vi "Intan_StreamData_128ch_parallelLoop_noEventStruct.vi"(0 "VISA resource name":refnum<visa-resource-name>, 1 "refnum in":refnum<file>, 3 "stop streaming":bool, 4 "Save Binary Data":bool, 5 "error in":errorcluster, 7 "byte order":T5(ring)=enum."little-endian", 8 "hdr fpath":path, 9 "MaxStreamChans":u16=32, 11 "DT_scale (sec)":dbl=0.01, 12 "aux file ref num":refnum<file>, 14 "save aux file":bool) -> (6 "N data scans to read (VISA)":i32=20, 10 "Nbytes VISA read":u32, 13 "VISA read iter":i32, 19 "error out":errorcluster)   [LabVIEW 2020]
doc: "Stream data to disk and user friendly display. Data is scaled and filtered prior to display.\n\nThis VI uses parallel while loop architecture: 1 loop reads from serial stream and saves raw bytes to disk; the other loop processes the data in chunk, scaling and filtering, then displays."
uses:
  zip_swcircularbuffer1_0_19b/Circular Buffer/Controls/Circular Buffer Status.ctl
  zip_swcircularbuffer1_0_19b/Circular Buffer/Controls/Circular Buffer Operations.ctl
  <vilib>/Utility/error.llb/DialogType.ctl
  <vilib>/Analysis/baseanly.llb/Mean (DBL).vi
  zip_swcircularbuffer1_0_19b/Circular Buffer/Instance VIs/Circular Buffer(1D U16).vi
  zip_swcircularbuffer1_0_19b/Circular Buffer/Circular Buffer.lvlib
  <vilib>/Analysis/NI_AALBase.lvlib
panel:
  out "A+B+C+D chans":i32[](array[numeric])
  out "C+D chans":i32[](array[numeric])
  out "Dchans":i32[](array[numeric])
  out "Cchans":i32[](array[numeric])
  out "ADXL/Vflex/Vdd Stream":dbl[][](graph)
  out "A+B chans":i32[](array[numeric])
  out "Bchans":i32[](array[numeric])
  out "Achans":i32[](array[numeric])
  in  "Tab Control":T1(tab)
  in  "Update Channels":bool
  in  "Accel/Vdd/Vflex":i32[](listbox)
  in  "stop logging":bool
  in  "DisplayScale (uV/div)":u16(ring)=1 items=["6400", "3200", "1600", "800", "400", "200", "100", "50", "25"]
  in  "offset factor":dbl=1.0
  in  "Filter settings":T2={"LP Filter On/Off"=TRUE, "LP Cutoff (Hz)"=40.0, "HP Filter On/Off"=TRUE, "HP Cutoff (Hz)"=0.5, "Bandstop On/Off"=TRUE, "fl Cutoff (Hz)"=48.0, "fh Cutoff (Hz) "=52.0}
  out "Save status":bool
  out "non integer read":bool
  out "display iter":i32
  out "% buffer full":dbl(slide) scale=0.0..100.0
  in  "Ring Buffer Size":T3={"Samples per Channel"=640000, "Channels"=0}
  out "buffer underflow":bool
  out "Buffer Status  (read)":T4
  out "buffer overflow":bool
  out "Buffer Status (write)":T4
  in  "Center Traces":bool
  in  "Amplifier Chans":i32[](listbox)=[1, 4, 13, 14, 15, 16, 17, 22]
  out "FS (Hz)":dbl
  in  "ChartDisplayLength (s)":dbl=5.0
  in  "Display Update interval (ms)":dbl=100.0
  in  "Buffer Read Interval (ms)":i16=100
  in  "ChanSelect":u16(ring)=7 items=["A chans (0-31)", "B chans (32-63)", "C chans (64-95)", "D chans (96-127)", "A+B chans (0-63)", "C+D chans (64-127)", "Free Select", "None"]
  out "Vdd amp (V)":dbl format="%0.1f"
  in  "bytes per data frame":i32=286
  in  "Nchans":i32=128
  in  "start stream (Teensy char)":string="s"
  in  "stop serial stream (Teensy char)":string="t"
  out "Text response":string
  out "aux_cmd_array":i32[][](array[numeric])
  out "binary data (from VISA read)":u16[](array[numeric])
  out "magicNum Out":i32[](array[numeric])
  in  "stop logging Teensy char":string="l"
  out "Vdd (V) out":dbl[](array[numeric])
  out "accel + flex + Vdd array":dbl[][](array[numeric])
  out "Vflex (V) out":dbl[](array[numeric])
  out "Data Frame Locked":string="circ buffer write:\nelement 0 ~= 73!"
  out "setscaleresult":dbl
  out "UpdateCode":i16
  out "xmax_init":dbl
  out "offset_init":dbl
  out "increment_init":dbl
  out "xmin_init":dbl
  out "NchansChanged":bool
  out "DispLengthChanged":bool
  out "XscaleRollover":bool
  out "error code out":i32 format="%0.0f"
  out "StopLoopsMaster":bool
  out "N_u16s  write to buf":i32
  out "Nelements to read from buf":dbl
  out "N data scans to display":u16=20
  out "YtxtLabelsAll":string[](array[string])
  out "bytes streaming per frame":u16
  out "requestBytes":dbl
  out "SerRead":string
  out "lengthCorStr":i32
  out "CorrectedSubstring":string
  out "NmissingFromFrame":i32
  out "bytesParsed":i32=148
  out "adxl size":i32[](array[numeric])
  out "intan size":i32[](array[numeric])
  out "ChanSelect(uint32)":u32[](array[numeric])
  out "ChanSelString":string
  out "NumChansNewStream":string
  out "Buffer Status Empty Buf":T4
  out "NumStreamingCluster":T6
  out "AmpsList":u16[](array[numeric])
  out "ClusterPropnod":T6
  out "ClusterLocalVar":T6
  out "Elements Remaining":i32
  out "termcharsReadBuffer":string
  out "termcharsCount":u32
  out "NumChansStreaming":i16
  out "initRead":string[](array[string])
  out "CircBufWrite":u16[](array[numeric])
  out "ReadCircBuf":u16[](array[numeric])
  out "subReadArray":u16[](array[numeric])
  out "corrected array":u16[](array[numeric])
  out "Nextraadded":i32
  out "extrareadelements":u16[](array[numeric])
  out "Picture":picture
  out "Intan Streaming Data":dbl[][](graph)
  # "Intan-Teensy Bioelectric Module: Data Stream and Visualization\n128 chan + ADXL"
  # "Data Streaming Frequency"
  # "Display Settings"
  # "Ring Buffer Status"
  # "1-D data stream \nreformatted  to 2-D"
  # "xscale controls"
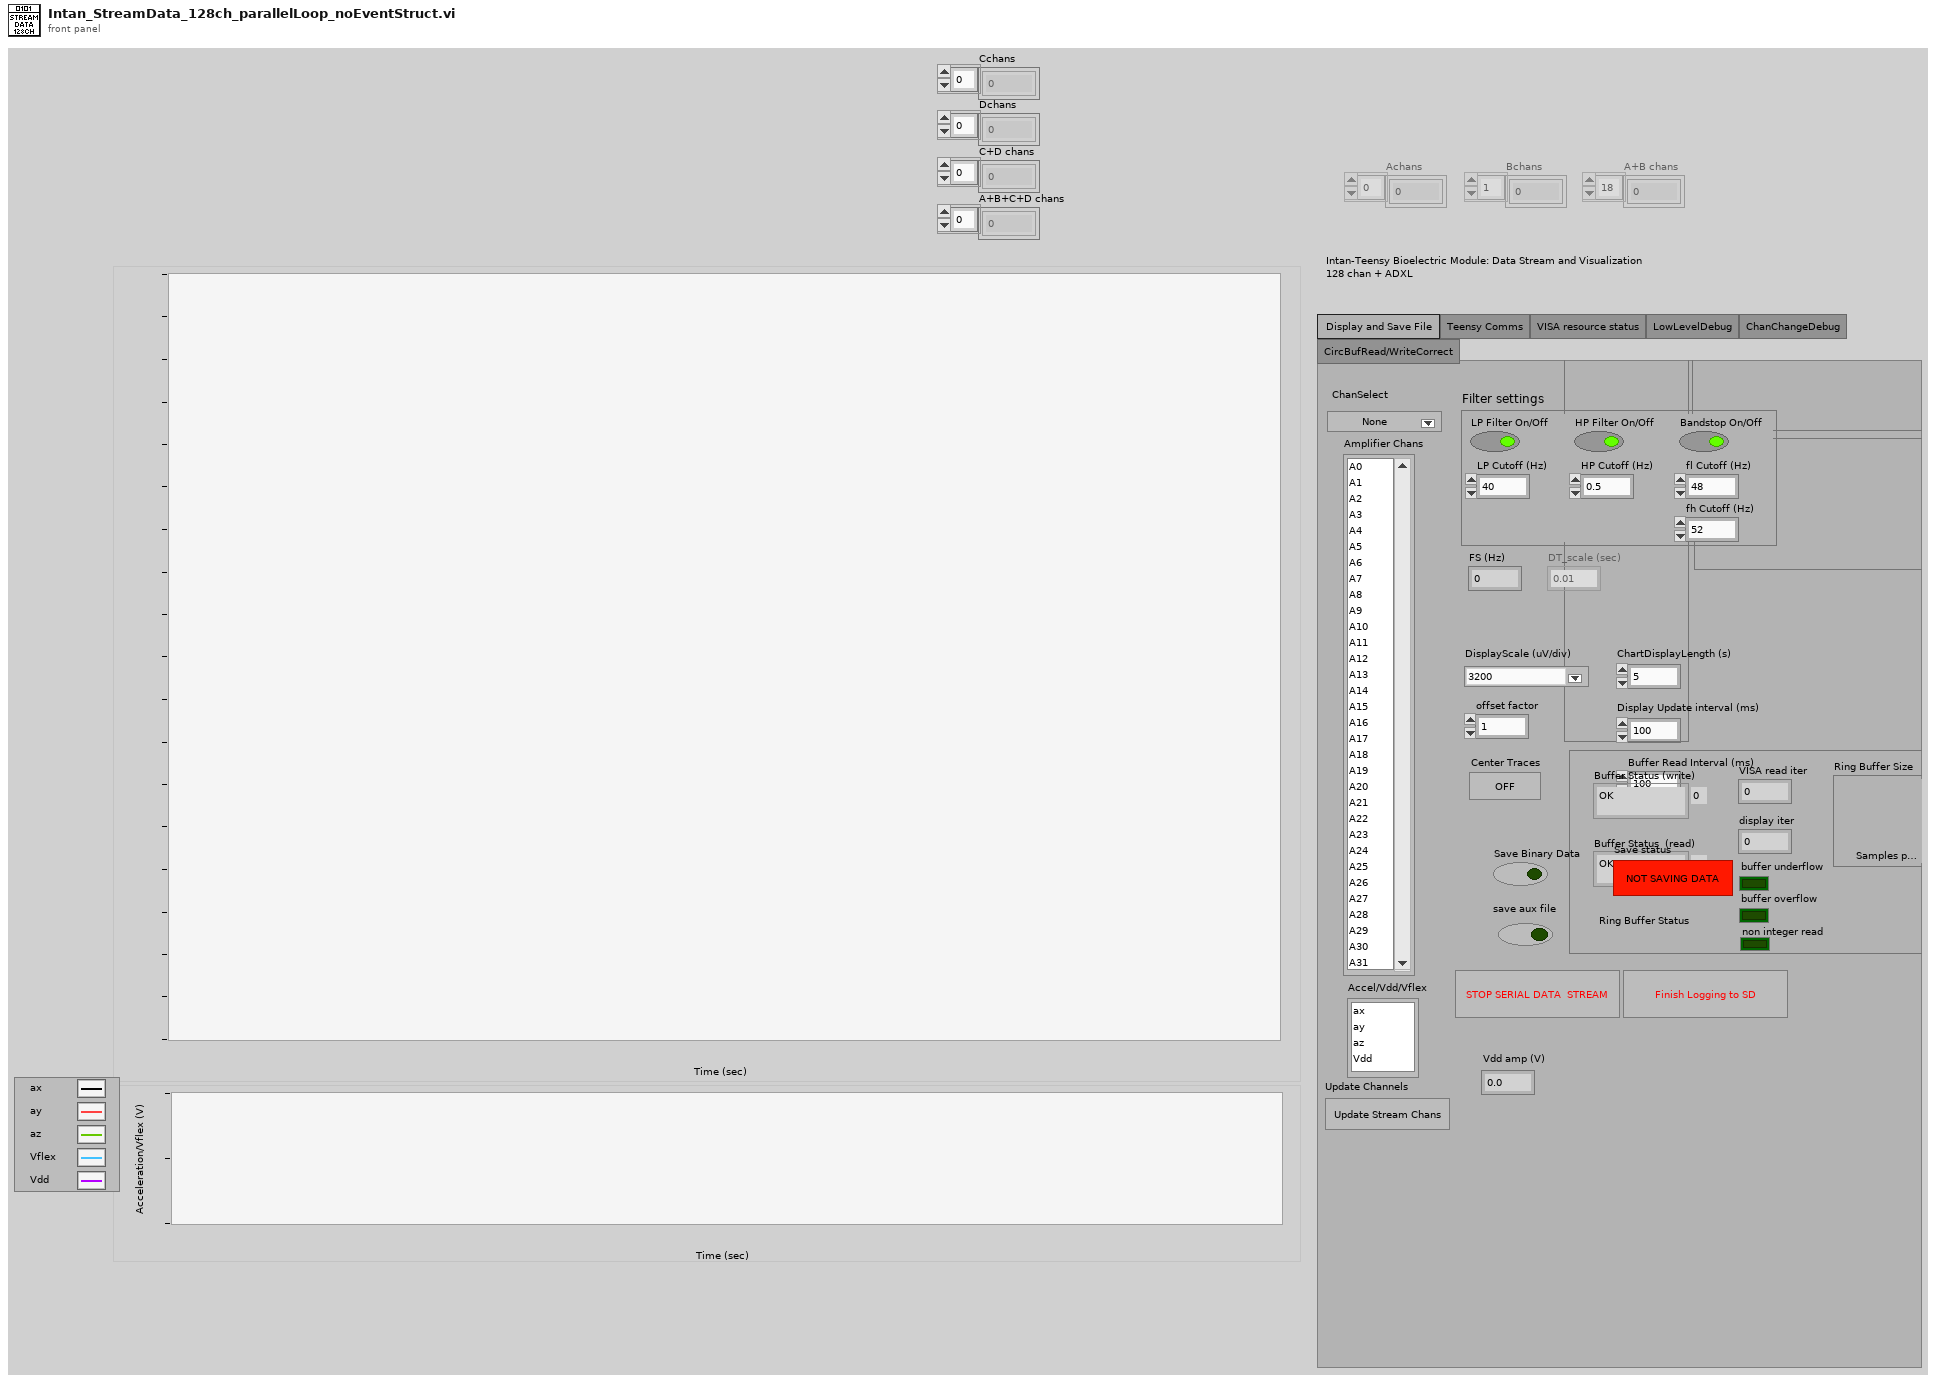
[diagram p1: front panel]
types:
  T1 = enum32{"Display and Save File ", "Teensy Comms", "VISA resource status", "LowLevelDebug", "ChanChangeDebug", "CircBufRead/WriteCorrect"}
  T2 = cluster{"LP Filter On/Off":bool, "LP Cutoff (Hz)":dbl, "HP Filter On/Off":bool, "HP Cutoff (Hz)":dbl, "Bandstop On/Off":bool, "fl Cutoff (Hz)":dbl, "fh Cutoff (Hz) ":dbl}
  T3 = cluster{"Samples per Channel":u32, "Channels":u32}
  T4 = typedef "Circular Buffer.lvlib/Circular Buffer Status.ctl" = enum16{"OK", "Overflow", "Underflow"}
  T5 = enum16{"big-endian, network order", "native, host order", "little-endian"}
  T6 = cluster{"NumChansStreaming":i16, "NumAmps":i32, "NumAccel":i32, "NumVdd":i32, "NumVflex":i32}
  T7 = enum8{"Enabled", "Disabled", "Disabled and Grayed Out"}
  T8 = typedef "Circular Buffer.lvlib/Circular Buffer Operations.ctl" = enum16{"Initialize", "Get Backlog", "Write", "Read (continuous)", "Read (most recent)"}
  T9 = typedef "LVRectTypeDef.ctl" = cluster{"Left":i16, "Top":i16, "Right":i16, "Bottom":i16}
  T10 = typedef "DialogType.ctl" = u16
  T11 = cluster{"XScale.Minimum":dbl, "XScale.Maximum":dbl, "XScale.Increment":dbl, "Nchannels":i32}
  T12 = cluster{"Maximum":dbl, dbl, dbl, dbl, dbl, dbl, "YscleMark":dbl, "Increment":dbl}
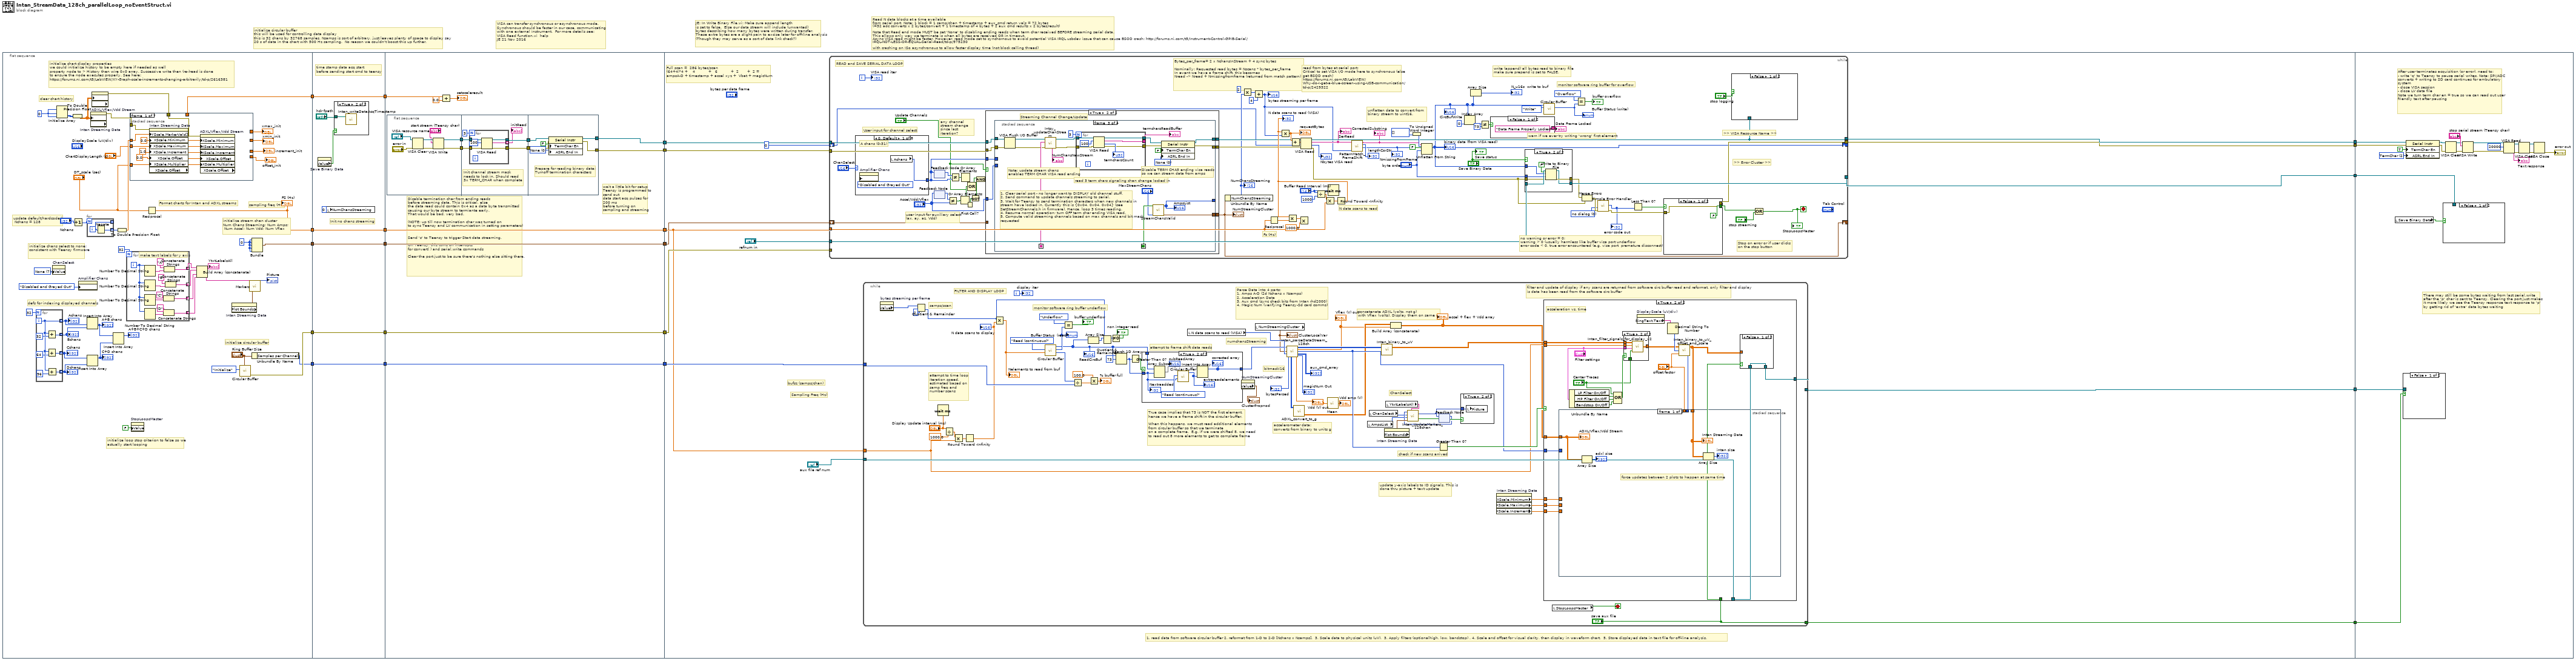
[diagram p0: block diagram]
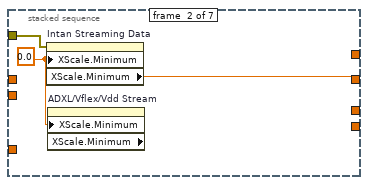
[diagram p2: hidden frame]
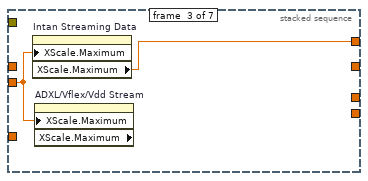
[diagram p3: hidden frame]
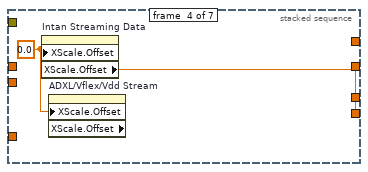
[diagram p4: hidden frame]
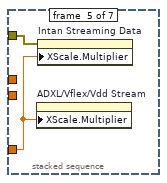
[diagram p5: hidden frame]
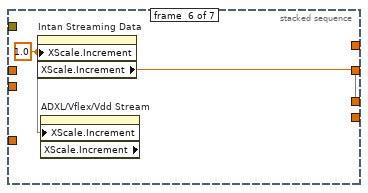
[diagram p6: hidden frame]
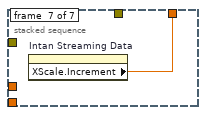
[diagram p7: hidden frame]
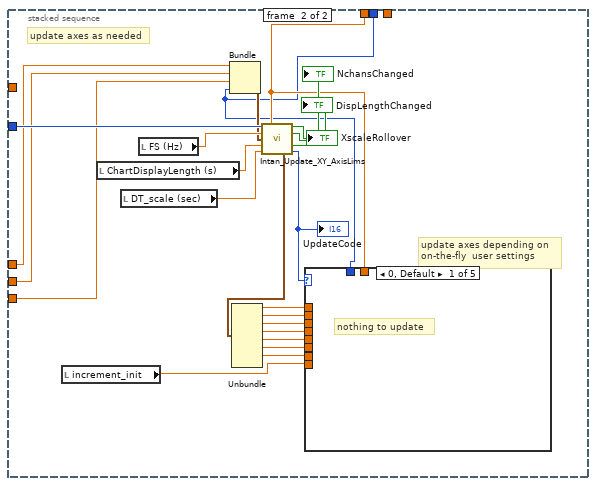
[diagram p12: hidden frame]
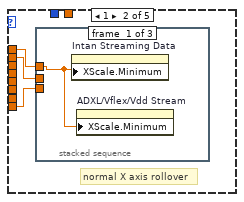
[diagram p13: hidden frame]
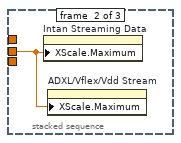
[diagram p14: hidden frame]
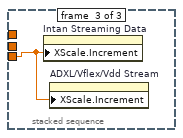
[diagram p15: hidden frame]
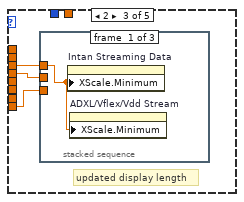
[diagram p16: hidden frame]
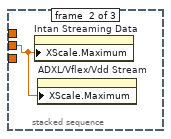
[diagram p17: hidden frame]
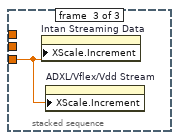
[diagram p18: hidden frame]
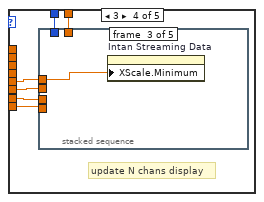
[diagram p19: hidden frame]
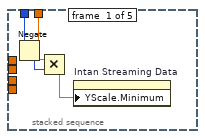
[diagram p20: hidden frame]
diagram:
  # "Read N data blocks at a time available\nfrom serial port. Note: 1 block = 1 samp/chan + timestamp + aux_cmd return vals = 72 bytes \n(=32 adc converts x 2 bytes/convert + 1 timestamp of 4 bytes + 2 aux cmd results x 2 bytes/result) \n\nNote that Read end mode MUST be set 'None' to disabling ending reads when term char received BEFORE streaming serial data.  \nThis allows only way we terminate is when all bytes are received OR in timeout.  \nAsync VISA read might be faster. However, read mode set to synchornous to avoid potential VISA IRQL usbdev issue that can cause BSOD crash: http://forums.ni.com/t5/Instrument-Control-GPIB-Serial/IRQL-NOT-LESS-OR-EQUAL-Serial-Read/td-p/975230\n\nwith crashing on ISo asynchronous to allow faster display time (not block calling thread)"
  # "initialize circular buffer\nthis will be used for controlling data display\nthis is 32 chans by 32768 samples. Nsamps is sort of arbitrary, just leaves plenty of space to display say\n20 s of data in the chart with 500 Hz sampling.  No reason we couldn't boost this up further."
  # "JE: In Write Binary File.vi: Make sure append length \nis set to false.  Else our data stream will include (unwanted)\nbytes describing how many bytes were written during transfer.\nThese extra bytes are a slight pain to excise later for off-line analysis\n(Though they may serve as a sort of data link check?)"
  # "VISA can transfer synchronous or asynchronous mode.\nSynchronous should be faster in our case, communicating\nwith one external instrument.  For more details see: \nVISA Read function.vi  help \nJE 21 Nov 2016"
  n1 = flat-sequence {
    tunnel: [w60] -> w13
    tunnel: [w58] -> w11
    tunnel: [w54] -> w9
    tunnel: [w43] -> w7
    tunnel: [w25] -> w5
    tunnel: w13 -> [w113]
    tunnel: [w113] -> w12
    tunnel: w11 -> [w112]
    tunnel: [w112] -> w10
    tunnel: w9 -> [w111]
    tunnel: [w111] -> w8
    tunnel: w7 -> [w110]
    tunnel: [w110] -> w6
    tunnel: w5 -> [w106]
    tunnel: [w106] -> w4
    tunnel: [w127] -> w19
    tunnel: w12 -> [w127]
    tunnel: [w126] -> w18
    tunnel: w10 -> [w126]
    tunnel: [w125] -> w17
    tunnel: w8 -> [w125]
    tunnel: w6 -> [w124]
    tunnel: w4 -> [w121]
    tunnel: [w121] -> w3
    tunnel: [w115] -> w2
    tunnel: [w116] -> w1
    tunnel: [w164] -> w21
    tunnel: [w165] -> w20
    tunnel: w19 -> [w163]
    tunnel: w18 -> [w162]
    tunnel: w17 -> [w161]
    tunnel: [w160] -> w16
    tunnel: [w158] -> w15
    tunnel: [w157] -> w14
    tunnel: w3 -> [w156]
    tunnel: w2 -> [w154]
    tunnel: w1 -> [w155]
    tunnel: w21 -> [w498]
    tunnel: w20 -> [w511]
    tunnel: w16 -> [w493]
    tunnel: w15 -> [w492]
    tunnel: w14 -> [w491]
    frame #0 {
      w24 = u16 7 items=["A chans (0-31)", "B chans (32-63)", "C chans (64-95)", "D chans (96-127)", "A+B chans (0-63)", "C+D chans (64-127)", "Free Select", "None"] ("ChanSelect")
      w22 = i16 0
      w53 = 0 ("Dimension Size")
      # "initialize chans select to none; consistent with Teensy firmware"
      # "initialize stream chan cluster\nNum Chans Streaming; Num Amps;\n Num Accel; Num Vdd; Num Vflex"
      # "initialize circular buffer"
      # "Format charts for Intan and ADXL streams"
      # "defs for indexing displayed channels"
      # "update default/hardcoded\n Nchans = 128"
      # "clear chart history"
      # "initialize loop stop criterion to false so we\nactually start looping"
      # "sampling freq (Hz)"
      # "initialize chart display properties\nwe could initialize history to be empty here if needed as well\nproperty node to > History then wire 0x0 array. Successive write then (re-)read is done\nto ensure the node executes properly. See here:\nhttps://forums.ni.com/t5/LabVIEW/XY-Graph-scale-increments-changing-arbitrarily/td-p/2616381"
      n2 = for {
        N: 32 -> [_]
        tunnel: [w68] -> w35 mode=indexing
        tunnel: [w69] -> w34 mode=indexing
        tunnel: [w65] -> w33 mode=indexing
        tunnel: [w64] -> w32 mode=indexing
        i -> [w68]
        n3 = Add(x=w68, y=32) -> (x+y=w69:i32)
        n4 = Add(x=w68, y=64) -> (x+y=w65:i32)
        n5 = Add(x=w68, y=96) -> (x+y=w64:i32)
      }
      "Achans" <- w35
      "Bchans" <- w34
      "Cchans" <- w33
      "Dchans" <- w32
      n6 = property on="ChanSelect" class="Ring (strict)"("Value"=w24) -> ()  [unwired: 2 in, 2 out]
      n7 = Initialize Array(w53, w53, w53) -> (w52:i32[][])
      n8 = To Double Precision Float(number=w52) -> (double precision float=w37:dbl[][])
      n9 = Increment(x="Nchans") -> (x+1=w62:i32)
      n10 = property on="Amplifier Chans" class="LstBox (strict)"("DisabledEnum"=T7."Disabled and Grayed Out" ("Disabled")) -> ()  [unwired: 2 in, 2 out]
      n11 = for {
        N: w62 -> [_]
        tunnel: [w105] -> w63 mode=indexing
        tunnel: [w104] -> _ mode=indexing
        i -> [w104]
        n12 = Negate(x=w104) -> (-x=w105:i32)
      }
      n13 = Insert Into Array(array=w35, new element=w34) -> (w31:i32[])  [unwired: 1 in]
      "A+B chans" <- w31
      n14 = Insert Into Array(array=w33, new element=w32) -> (w30:i32[])  [unwired: 1 in]
      "C+D chans" <- w30
      n15 = property on="Intan Streaming Data" class="WFChart (strict)" props=["History Data", "History Data"]("History Data"=w37) -> (error out=w50:errorcluster)  [unwired: 2 in, 2 out]
      n16 = property on="ADXL/Vflex/Vdd Stream" class="WFChart (strict)" props=["History Data", "History Data"]("History Data"=w37) -> (error out=w36:errorcluster)  [unwired: 2 in, 2 out]
      n17 = Insert Into Array(array=w31, new element=w30) -> (→"A+B+C+D chans":i32[])  [unwired: 1 in]
      n18 = To Double Precision Float(number=w63) -> (double precision float=w51:dbl[])
      n19 = for {
        N: 32 -> [_]
        tunnel: [w101] -> w40 mode=indexing
        tunnel: [w98] -> w39 mode=indexing
        tunnel: [w92] -> w28 mode=indexing
        tunnel: [w91] -> w27 mode=indexing
        i -> [w97]
        # "make text labels for y axis"
        n20 = Number To Decimal String(number=w97) -> (decimal integer string=w103:string)  [unwired: 1 in]
        n21 = Number To Decimal String(number=w97) -> (decimal integer string=w100:string)  [unwired: 1 in]
        n22 = Number To Decimal String(number=w97) -> (decimal integer string=w93:string)  [unwired: 1 in]
        n23 = Number To Decimal String(number=w97) -> (decimal integer string=w94:string)  [unwired: 1 in]
        n24 = Concatenate Strings("D" ("string"), w94) -> (w91:string)
        n25 = Concatenate Strings("C" ("string"), w93) -> (w92:string)
        n26 = Concatenate Strings("A" ("string"), w103) -> (w101:string)
        n27 = Concatenate Strings("B" ("string"), w100) -> (w98:string)
      }
      n28 = stacked-sequence {
        tunnel: w51 -> [w78 _ _ _ _ _ _]
        tunnel: w50 -> [w77 w80 _ _ w87 _ _]
        tunnel: "ChartDisplayLength (s)" -> [w75 _ w82 _ _ _ _]
        tunnel: "DT_scale (sec)" -> [w72 _ _ _ w86 _ _]
        tunnel: [_ _ w83 _ _ _ _] -> w44
        tunnel: [_ w81 _ _ _ _ _] -> w47
        tunnel: [_ _ _ _ _ w89 _] -> w46
        tunnel: [_ _ _ w85 _ _ _] -> w45
        tunnel: [_ _ _ _ _ _ w90] -> w43
        tunnel: w36 -> [w71 _ _ _ _ _ _]
        frame #0 {
          w74 = 1.0 ("X Scale.Range:Minimum")
          w73 = 0.0 ("X Scale.Range:Minimum")
          w76 = 0.0 ("X Scale.Range:Minimum")
          n29 = property on="Intan Streaming Data" class="WFChart (strict)" props=["YScale", "MarkerVals[]", "XScale", "Minimum", "XScale", "Maximum", "XScale", "Increment", "XScale", "Offset", "XScale", "Multiplier", "XScale", "Offset"](error in=w77, "YScale.MarkerVals[]"=w78, "XScale.Minimum"=w76, "XScale.Maximum"=w75, "XScale.Increment"=w74, "XScale.Offset"=w73, "XScale.Multiplier"=w72) -> ()  [unwired: 1 in, 3 out]
          n30 = property on="ADXL/Vflex/Vdd Stream" class="WFChart (strict)" props=["XScale", "Minimum", "XScale", "Maximum", "XScale", "Increment", "XScale", "Offset", "XScale", "Multiplier", "XScale", "Offset"](error in=w71, "XScale.Minimum"=w76, "XScale.Maximum"=w75, "XScale.Increment"=w74, "XScale.Offset"=w73, "XScale.Multiplier"=w72) -> ()  [unwired: 1 in, 3 out]
        }
        frame #1 {
          w79 = 0.0 ("X Scale.Range:Minimum")
          n31 = property on="Intan Streaming Data" class="WFChart (strict)"(error in=w80, "XScale.Minimum"=w79) -> ("XScale.Minimum"=w81:dbl)  [unwired: 1 in, 2 out]
          n32 = property on="ADXL/Vflex/Vdd Stream" class="WFChart (strict)" props=["XScale", "Minimum", "XScale", "Minimum"]("XScale.Minimum"=w79) -> ()  [unwired: 2 in, 3 out]
        }
        frame #2 {
          n33 = property on="Intan Streaming Data" class="WFChart (strict)"("XScale.Maximum"=w82) -> ("XScale.Maximum"=w83:dbl)  [unwired: 2 in, 2 out]
          n34 = property on="ADXL/Vflex/Vdd Stream" class="WFChart (strict)" props=["XScale", "Maximum", "XScale", "Maximum"]("XScale.Maximum"=w82) -> ()  [unwired: 2 in, 3 out]
        }
        frame #3 {
          w84 = 0.0 ("X Scale.Offset and Multiplier:Offset")
          n35 = property on="Intan Streaming Data" class="WFChart (strict)"("XScale.Offset"=w84) -> ("XScale.Offset"=w85:dbl)  [unwired: 2 in, 2 out]
          n36 = property on="ADXL/Vflex/Vdd Stream" class="WFChart (strict)" props=["XScale", "Offset", "XScale", "Offset"]("XScale.Offset"=w84) -> ()  [unwired: 2 in, 3 out]
        }
        frame #4 {
          n37 = property on="ADXL/Vflex/Vdd Stream" class="WFChart (strict)"("XScale.Multiplier"=w86) -> ()  [unwired: 2 in, 2 out]
          n38 = property on="Intan Streaming Data" class="WFChart (strict)"(error in=w87, "XScale.Multiplier"=w86) -> ()  [unwired: 1 in, 2 out]
        }
        frame #5 {
          w88 = 1.0 ("X Scale.Range:Increment")
          n39 = property on="Intan Streaming Data" class="WFChart (strict)"("XScale.Increment"=w88) -> ("XScale.Increment"=w89:dbl)  [unwired: 2 in, 2 out]
          n40 = property on="ADXL/Vflex/Vdd Stream" class="WFChart (strict)" props=["XScale", "Increment", "XScale", "Increment"]("XScale.Increment"=w88) -> ()  [unwired: 2 in, 3 out]
        }
        frame #6 {
          n41 = property on="Intan Streaming Data" class="WFChart (strict)"() -> ("XScale.Increment"=w90:dbl)  [unwired: 2 in, 2 out]
        }
      }
      "xmin_init" <- w47
      "increment_init" <- w46
      "offset_init" <- w45
      "xmax_init" <- w44
      n42 = property on="StopLoopsMaster" class="Bool (strict)"("Value"=FALSE ("StopLoopsMaster")) -> ()  [unwired: 2 in, 2 out]
      n43 = Reciprocal(x="DT_scale (sec)") -> (1/x=w54:dbl)
      "FS (Hz)" <- w54
      n44 = Build Array (concatenate)(w40, w39, w28, w27) -> (w38:string[])
      "YtxtLabelsAll" <- w38
      n45 = property on="Intan Streaming Data" class="WFChart (strict)"() -> ("Plot Bounds"=w55:T9)  [unwired: 2 in, 2 out]
      n46 = call-poly "Circular Buffer.vi"("Buffer Size"="Ring Buffer Size", "Operation"=Circular_Buffer_Operations."Initialize") -> ("error out"=w60:errorcluster)  [unwired: 6 in, 3 out]
      n47 = call "Markers.vi"("plot bounds"=w55, "Array"=w38) -> ("Picture"=→"Picture":picture)  [unwired: 1 out]
      n48 = Bundle(w22, w22, w22, w22, w22) -> (w25:cluster{i16, i16, i16, i16, i16})  [unwired: 1 in]
      n49 = Unbundle By Name("Ring Buffer Size") -> ("Samples per Channel"=w58:u32)
    }
    frame #1 {
      # "Init no chans streaming"
      # "time stamp data acq start\nbefore sending start cmd to teensy"
      n50 = property on="Save Binary Data" class="Bool (strict)"() -> ("Value"=w109:bool)  [unwired: 2 in, 2 out]
      n51 = local write "NumChansStreaming"(i16 0 ("NumChansStreaming")) -> ()
      n52 = case shown="True" w109 {
        tunnel: "hdr fpath" -> [_ w114]
        frame False {
        }
        frame True {
          n53 = call "Intan_writeDataAcqTimestamp.vi"("hdr fpath"=w114) -> ()  [unwired: 2 in, 1 out]
        }
      }
    }
    frame #2 {
      # "wait a little bit for setup\nTeensy is programmed to send out \ndata start acq pulses for 200 ms\nbefore turning on sampling and streaming"
      # "Disable termination char from ending reads\nbefore streaming data. This is critical, else\nthe data read could contain 0x4 as a data byte transmitted\ncausing our byte stream to termiante early.\nThat would be bad, very bad.\n\n(NOTE: up till now termination char was turned on\nto sync Teensy and LV communication in setting parameters)\n\n\nSend 's' to Teensy to trigger Start data streaming.  \n\nOn Teensy, this turns on interrupts\nfor convert( ) and serial.write commands\n\nClear the port just to be sure there's nothing else sitting there."
      n54 = flat-sequence {
        tunnel: [w129] -> w118
        tunnel: [w128] -> w117
        tunnel: [w136] -> w120
        tunnel: [w137] -> w119
        tunnel: w118 -> [w139]
        tunnel: w117 -> [w138]
        tunnel: w120 -> [w149]
        tunnel: w119 -> [w150]
        tunnel: [w148] -> w116
        tunnel: [w147] -> w115
        frame #0 {
          n55 = VISA Clear(VISA resource name="VISA resource name", error in (no error)="error in") -> (VISA resource name out=w132:refnum<visa-resource-name>, error out=w131:errorcluster)
          n56 = VISA Write(VISA resource name=w132, write buffer="start stream (Teensy char)", error in (no error)=w131) -> (VISA resource name out=w129:refnum<visa-resource-name>, error out=w128:errorcluster)  [unwired: 1 out]
        }
        frame #1 {
          # "Init channel stream mask\nneeds to lock in. Should read\n3x TERM_CHAR when complete"
          n57 = for {
            N: 3 -> [_]
            tunnel: w139 -> [w146]
            tunnel: w138 -> [w145]
            tunnel: [w143] -> w137
            tunnel: [w142] -> w136
            tunnel: [w141] -> w135 mode=indexing
            n58 = VISA Read(VISA resource name=w146, byte count=u32 100, error in (no error)=w145) -> (VISA resource name out=w143:refnum<visa-resource-name>, read buffer=w141:string, error out=w142:errorcluster)  [unwired: 1 out]
          }
          "initRead" <- w135
        }
        frame #2 {
          w151 = u16 0 items=["None", "Last Bit", "TermChar"] ("Serial Settings:End Mode for Reads")
          # "Prepare for reading binary data; \nTurnoff termination characters"
          n59 = property class="Serial Instr"(reference=w150, error in=w149, "TermChar En"=FALSE ("Message Based Settings:Termination Character Enable"), "ASRL End In"=w151) -> (reference out=w148:refnum<visa-resource-name>, error out=w147:errorcluster)
        }
      }
      n60 = Add(x=w124, y=0.0) -> (x+y=→"setscaleresult":dbl)
    }
    frame #3 {
      # "Sampling Freq (Hz)"
      # "Full scan =  286 bytes/scan\n(64+4)*4 +    4           +   6           +  2       +  2 =\nampsA-D + timestamp + accel xyz +  Vbat + magicNum"
      # "1. read data from software circular buffer 2. reformat from 1-D to 2-D [Nchans x Nsamps].  3. Scale data to physical units (uV).  3. Apply filters (optionalhigh, low, bandstop) . 4. Scale and offset for visual clarity, then display in waveform chart.  5. Store displayed data in text file for off-line analysis."
      # "bufsz (samps/chan)"
      n61 = while {
        tunnel: [w372] -> w164
        tunnel: [w406] -> w165
        tunnel: "refnum in" -> [w405]
        tunnel: w163 -> [_]
        tunnel: w161 -> [w375]
        tunnel: [w379] -> w158
        shift-right: [w348] -> _
        shift-left: w156 -> [w356]
        tunnel: w155 -> [w355]
        tunnel: w154 -> [w354]
        shift-right: [w343] -> _
        shift-left: 0 ("NmissingFromFrame") -> [w341]
        i -> [w404]
        stop <- w407 stop-if-true
        w385 = T10 0 items=["no dialog", "OK message", "continue or stop message", "OK message + warnings", "continue/stop + warnings"] ("type of dialog (OK msg:1)")
        # "warn if we ever try writing 'wrong' first element"
        # "user input for auxiliary select\n(ax, ay, az, Vdd)"
        # "User input for channel select"
        # "any channel stream change since last iteration?"
        # "Bytes_per_frame= 2 x NchansInStream + 4 sync bytes\n\nNominally: Requested read bytes = Nscans * bytes_per_frame\nIn event we have a frame shift, this becomes \nNread -> Nread + Nmissingfromframe (returned from match pattern)"
        # "N data scans to read"
        # "Fs (Hz)"
        # "no warning or error = 0;\nwarning > 0 (usually harmless like buffer visa port underflow\nerror code < 0, true error encountered (e.g. visa port  premature disconnect)"
        # "READ and SAVE SERIAL DATA LOOP"
        # "monitor software ring buffer for overflow"
        # "write (append) all bytes read to binary file\nmake sure prepend is set to FALSE."
        # "unflatten data to convert from binary stream to uint16."
        # "Stop on error or if user clicks \non the stop button"
        # ">> Error Cluster >>"
        # ">> VISA Resource Name >>"
        # "read from bytes at serial port:\nCritical to set VISA I/O mode here to synchronous (else get BSOD crash)\nhttps://forums.ni.com/t5/LabVIEW/Why-do-I-get-a-blue-screen-using-USB-communication/td-p/2429322"
        n62 = case shown="0, Default" "ChanSelect" {
          tunnel: [w456 w458 w460 w462 w464 w466 "Amplifier Chans" w470] -> w367
          frame 0, Default {
            # "A chans (0-31)"
            n63 = property on="Amplifier Chans" class="LstBox (strict)"("DisabledEnum"=T7."Disabled and Grayed Out" ("Disabled")) -> ()  [unwired: 2 in, 2 out]
            n64 = local read "Achans"() -> (w456:i32[])
          }
          frame 1 {
            # "B chans (32-63)"
            n65 = property on="Amplifier Chans" class="LstBox (strict)"("DisabledEnum"=T7."Disabled and Grayed Out" ("Disabled")) -> ()  [unwired: 2 in, 2 out]
            n66 = local read "Bchans"() -> (w458:i32[])
          }
          frame 2 {
            # "C chans (64-95)"
            n67 = property on="Amplifier Chans" class="LstBox (strict)"("DisabledEnum"=T7."Disabled and Grayed Out" ("Disabled")) -> ()  [unwired: 2 in, 2 out]
            n68 = local read "Cchans"() -> (w460:i32[])
          }
          frame 3 {
            # "D chans (96-127)"
            n69 = property on="Amplifier Chans" class="LstBox (strict)"("DisabledEnum"=T7."Disabled and Grayed Out" ("Disabled")) -> ()  [unwired: 2 in, 2 out]
            n70 = local read "Dchans"() -> (w462:i32[])
          }
          frame 4 {
            # "A and B chans (0-63)"
            # "no need to grab a subset"
            n71 = property on="Amplifier Chans" class="LstBox (strict)"("DisabledEnum"=T7."Disabled and Grayed Out" ("Disabled")) -> ()  [unwired: 2 in, 2 out]
            n72 = local read "A+B chans"() -> (w464:i32[])
          }
          frame 5 {
            # "C and D chans (64-127)"
            # "no need to grab a subset"
            n73 = property on="Amplifier Chans" class="LstBox (strict)"("DisabledEnum"=T7."Disabled and Grayed Out" ("Disabled")) -> ()  [unwired: 2 in, 2 out]
            n74 = local read "C+D chans"() -> (w466:i32[])
          }
          frame 6 {
            # "Free select"
            n75 = property on="Amplifier Chans" class="LstBox (strict)"("DisabledEnum"=T7."Enabled" ("Disabled")) -> ()  [unwired: 2 in, 2 out]
          }
          frame 7 {
            # "None"
            n76 = Initialize Array(i16 0 ("element"), 0 ("dimension size")) -> (w470:i16[])
          }
        }
        n77 = feedback #1() -> (w363:i32[])  [unwired: 1 in]
        n78 = feedback-in #1("Accel/Vdd/Vflex") -> ()
        n79 = feedback #2() -> (w366:i32[])  [unwired: 1 in]
        n80 = feedback-in #2(w367) -> ()
        n81 = Not Equal?(x=w363, y="Accel/Vdd/Vflex") -> (x != y?=w362:bool[])
        n82 = Not Equal?(x=w366, y=w367) -> (x != y?=w368:bool[])
        n83 = Or Array Elements(Boolean array=w362) -> (logical OR=w360:bool)
        n84 = Or Array Elements(Boolean array=w368) -> (logical OR=w361:bool)
        n85 = First Call?() -> (First Call?: T/F=w353:bool)
        n86 = Compound Arithmetic op=OR(w361, w360, "Update Channels") -> (w359:bool)
        n87 = Not(x=w353) -> (.not. x?=w350:bool)
        n88 = And(x=w359, y=w350) -> ()  [unwired: 1 out]
        n89 = case shown="True" "Update Channels" {
          tunnel: w367 -> [_ w419]
          tunnel: w355 -> [w411 w417]
          tunnel: [w411 w418] -> w365
          tunnel: w354 -> [w410 w416]
          tunnel: [w410 w415] -> w364
          tunnel: "Accel/Vdd/Vflex" -> [_ w414]
          tunnel: [w412 w413] -> w348
          tunnel: w356 -> [w412 _]
          frame False {
            # "no channel change requested since last loop iteration"
          }
          frame True {
            # "Streaming Channel Change/Update"
            n90 = stacked-sequence {
              seq-local: [w423 _ _ _] -> [_ _ w444 _]
              seq-local: [w421 _ _ _] -> [_ _ w447 _]
              tunnel: w419 -> [w424 _ _ _]
              tunnel: [_ _ w445 _] -> _
              tunnel: w417 -> [_ _ w442 _]
              tunnel: [_ _ w436 _] -> w418
              tunnel: w416 -> [_ _ w441 _]
              tunnel: [_ _ w435 _] -> w415
              tunnel: w414 -> [w420 _ _ _]
              tunnel: [_ _ w433 _] -> w413
              frame #0 {
                # "bitmask requested"
                # "configure 5 uint32 comma sep string"
                n91 = call "Intan_SetStreamChans.vi"("Amplifier Chans"=w424, "Accel/Vbat"=w420) -> ("ChanSelect(uint32)"=→"ChanSelect(uint32)":u32[], "ChanSelString"=w423:string, "BitMaskAll"=w421:bool[])
                "ChanSelString" <- w423
              }
              frame #1 {
                # "we don't need to visualize any of the samples that may be waiting/backlogged in circular buffer, read them all out, basically emptying the buffer to reset it"
                n92 = call-poly "Circular Buffer.vi"("Operation"=Circular_Buffer_Operations."Get Backlog") -> ("Elements Remaining"=→"Elements Remaining":i32, "Buffer Status"=→"Buffer Status Empty Buf":T4)  [unwired: 7 in, 2 out]
              }
              frame #2 {
                w438 = u16 0 items=["None", "Last Bit", "TermChar"] ("Serial Settings:End Mode for Reads")
                # "read 3 term chars signaling chan change locked in"
                # "Note: update stream chans\nenables TERM CHAR VISA read ending"
                # "Disable TERM CHAR ending visa reads\nso we can stream data from amps"
                # "1. Clear serial port - no longer want to DISPLAY old channel stuff.\n2. Send command to update channels streaming to serial.\n3. Wait for Teensy to send termination characters when new channels in stream have locked in. Currently this is {0x04, 0x04, 0x04} (see SetStreamChannels.h in firmware). Hence, loop 3 times reading. \n4. Resume normal operation; turn OFF term char ending VISA read.\n5. Compute valid streaming channels based on max channels and bit mask requested"
                n93 = VISA Flush I/O Buffer(VISA resource name=w442, error in (no error)=w441) -> (VISA resource name out=w430:refnum<visa-resource-name>, error out=w429:errorcluster)  [unwired: 1 in]
                n94 = call "Intsy_updateChanStream.vi"("error in (no error)"=w429, "ChanSelString"=w444, "VISA resource name"=w430) -> ("error out"=w432:errorcluster, "VISA resource name out"=w431:refnum<visa-resource-name>, "NStreamChansString"=→"NumChansNewStream":string)  [unwired: 5 in, 1 out]
                n95 = for {
                  N: 3 -> [_]
                  tunnel: w431 -> [w454]
                  tunnel: [w451] -> w437
                  tunnel: w432 -> [w450]
                  tunnel: [w449] -> w434
                  tunnel: [w448] -> w428
                  n96 = VISA Read(VISA resource name=w454, byte count=u32 100, error in (no error)=w450) -> (VISA resource name out=w451:refnum<visa-resource-name>, read buffer=w448:string, return count=→"termcharsCount":u32, error out=w449:errorcluster)
                }
                "termcharsReadBuffer" <- w428
                n97 = call "StreamChansValid.vi"("BitMaskRequested"=w447, "MaxStreamChans"="MaxStreamChans") -> ("AmpsList"=w445:u16[], "NumStreamingCluster"=w433:T6)  [unwired: 7 in, 5 out]
                "AmpsList" <- w445
                n98 = property class="Serial Instr"(reference=w437, error in=w434, "TermChar En"=FALSE ("Message Based Settings:Termination Character Enable"), "ASRL End In"=w438) -> (reference out=w436:refnum<visa-resource-name>, error out=w435:errorcluster)
              }
              frame #3 {
                # "reset channels button"
                n99 = local write "Update Channels"(FALSE ("Update Channels")) -> ()
              }
            }
          }
        }
        "NumStreamingCluster" <- w348
        n100 = Unbundle By Name(w348) -> ("NumChansStreaming"=w357:i16)
        "NumChansStreaming" <- w357
        n101 = Multiply(x=u16 2 ("y"), y=w357) -> (x*y=w370:u16)
        n102 = Add(x=w370, y=u16 4) -> (x+y=w345:u16)
        "bytes streaming per frame" <- w345
        n103 = Reciprocal(x=w375) -> (1/x=w389:dbl)
        n104 = Divide(x="Buffer Read Interval (ms)", y=i16 1000) -> (x/y=w377:dbl)
        n105 = Multiply(x=w377, y=w375) -> (x*y=w378:dbl)
        n106 = Wait (ms)(milliseconds to wait="Buffer Read Interval (ms)") -> ()  [unwired: 1 out]
        n107 = Round Toward -Infinity(1:w378) -> (0:w374:dbl)
        "N data scans to read (VISA)" <- w374
        n108 = Multiply(x=w374, y=w345) -> (x*y=w392:dbl)
        "requestBytes" <- w392
        n109 = Multiply(x=w374, y=w389) -> (x*y=w391:dbl)
        n110 = Add(x=w392, y=w341) -> (x+y=w342:dbl)
        n111 = Multiply(x=w391, y=1000.0) -> ()  [unwired: 1 out]
        n112 = VISA Read(VISA resource name=w365, byte count=w342, error in (no error)=w364) -> (VISA resource name out=w372:refnum<visa-resource-name>, read buffer=w347:string, return count=→"Nbytes VISA read":u32, error out=w387:errorcluster)
        "SerRead" <- w347
        n113 = call "PatternMatch_FrameShift.vi"("SerRead"=w347, "StreamingBytesPerFrame"=w345) -> ("OutputStr"=w344:string, "lengthCorr"=→"lengthCorStr":i32, "NmissingFromFrame"=w343:i32)  [unwired: 2 in, 3 out]
        "CorrectedSubstring" <- w344
        "NmissingFromFrame" <- w343
        n114 = To Unsigned Word Integer(number=i16[] []) -> (unsigned 16bit integer=w400:u16[])
        n115 = Unflatten From String(type=w400, binary string=w344, data includes array or string size? (T)=FALSE, byte order (0:big-endian, network order)="byte order") -> (value=w340:u16[])  [unwired: 1 in, 2 out]
        "binary data (from VISA read)" <- w340
        "CircBufWrite" <- w340
        n116 = Index Array(array=w340, index=0) -> (element=w338:u16)
        n117 = Array Size(array=w340) -> (size(s)=→"N_u16s  write to buf":i32)
        n118 = Not Equal?(x=w338, y=u16 73) -> (x != y?=w336:bool)
        n119 = case shown="False" w336 {
          tunnel: ["Data Frame Properly Locked" "circ buffer write:\nelement 0 ~= 73!" ("message")] -> w335
          frame False {
          }
          frame True {
          }
        }
        "Data Frame Locked" <- w335
        n120 = case shown="True" "Save Binary Data" {
          tunnel: [w482 w489] -> w388
          tunnel: [w481 w488] -> w406
          tunnel: w405 -> [w481 w487]
          tunnel: w387 -> [w482 w486]
          tunnel: "byte order" -> [_ w484]
          tunnel: w340 -> [_ w483]
          frame False {
          }
          frame True {
            n121 = Write to Binary File(file (use dialog)=w487, data=w483, error in=w486, 5:FALSE ("prepend array or string size? (T)"), 9:w484) -> (refnum out=w488:refnum<file>, error out=w489:errorcluster)  [unwired: 1 in, 1 out]
          }
        }
        n122 = call-poly "Circular Buffer.vi"("Operation"=Circular_Buffer_Operations."Write", "Data In"=w340) -> ("Buffer Status"=w395:T4)  [unwired: 6 in, 3 out]
        "Buffer Status (write)" <- w395
        n123 = Equal?(x=Circular_Buffer_Status."Overflow" ("y"), y=w395) -> (x = y?=→"buffer overflow":bool)
        n124 = Merge Errors(w388, w387) -> (w386:errorcluster)
        n125 = call <vilib>:"Simple Error Handler.vi"("type of dialog (OK msg:1)"=w385, "error in (no error)"=w386) -> ("code out"=w382:i32, "error out"=w383:errorcluster)  [unwired: 3 in, 3 out]
        "error code out" <- w382
        n126 = Less Than 0?(x=w382) -> (x < 0?=w380:bool)
        n127 = case shown="False" w380 {
          tunnel: w383 -> [w475 w479]
          tunnel: [FALSE TRUE] -> w381
          tunnel: [w475 w477] -> w379
          frame False {
          }
          frame True {
            n128 = call <vilib>:"Clear Errors.vi"("error in (no error)"=w479) -> ("error out"=w477:errorcluster)  [unwired: 5 in, 1 out]
            n129 = One Button Dialog(message=" stop loop, attempt graceful exit\nvisa read error") -> ()  [unwired: 1 in, 1 out]
          }
        }
        n130 = case shown="False" "stop logging" {
          tunnel: w372 -> [_ w474]
          frame False {
          }
          frame True {
            # "turns off SD logging"
            n131 = VISA Write(VISA resource name=w474, write buffer="stop logging Teensy char") -> ()  [unwired: 1 in, 3 out]
          }
        }
        n132 = Compound Arithmetic op=OR(w381, "stop streaming") -> (w407:bool)
        "StopLoopsMaster" <- w407
        "VISA read iter" <- w404
        "Save status" <- "Save Binary Data"
      }
      n133 = while {
        tunnel: w162 -> [w219]
        tunnel: w161 -> [w198]
        tunnel: [w203] -> w160
        tunnel: "aux file ref num" -> [w202]
        tunnel: ["save aux file"] -> w157
        i -> [w214]
        stop <- w200 stop-if-true
        # "concatenate ADXL (volts, not g)\nwith Vflex (volts). Display them on same axis"
        # "True case implies that 73 is NOT the first element, \nhence we have a frame shift in the circular buffer.\n\nWhen this happens, we must read additional elements from circular buffer so that we terminate \non a complete frame.  E.g. if we were shifted 8, we need\nto read out 8 more elements to get to complete frame"
        # "attempt to frame shift data reads"
        # "ChanSelect"
        # "bitmaskI16"
        # "numchansStreaming"
        # "samps/scan"
        # "accelerometer data: \nconverts from binary to units g"
        # "Parse Data into 4 parts:\n1. Amps A-D (2d Nchans x Nsamps) \n2. Acceleration Data\n3. Aux cmd (sync check bits from Intan rhd2000)\n4. Magic Num (verifying Teensy-Sd card comms)"
        # "check if new scans arrived"
        # "update y-axis labels to ID signals. This is done thru picture + text update"
        # "FILTER AND DISPLAY LOOP"
        # "attempt to time loop iteration speed,\nestimated based on samp freq and number scans"
        # "filter and update of display if any scans are returned from software circ buffer read and reformat. only filter and display is data has been read from the software circ buffer"
        # "monitor software ring buffer underflow"
        n134 = property on="bytes streaming per frame" class="DigNum (strict)"() -> ("Value"=w177:u16)  [unwired: 2 in, 2 out]
        n135 = Quotient & Remainder(x=w177, y=i16 2) -> (floor(x/y)=w183:u16)  [unwired: 1 out]
        n136 = Wait (ms)(milliseconds to wait="Display Update interval (ms)") -> ()  [unwired: 1 out]
        n137 = Divide(x="Display Update interval (ms)", y=1000.0) -> (x/y=w195:dbl)
        n138 = Multiply(x=w195, y=w198) -> (x*y=w197:dbl)
        n139 = Round Toward -Infinity(1:w197) -> (0:w196:dbl)
        "N data scans to display" <- w196
        n140 = Multiply(x=w183, y=w196) -> (x*y=w213:dbl)
        "Nelements to read from buf" <- w213
        n141 = call-poly "Circular Buffer.vi"("Read Size"=w213, "Operation"=Circular_Buffer_Operations."Read (continuous)") -> ("Elements Remaining"=w220:i32, "Buffer Status"=w222:T4, "Data Out"=w173:u16[])  [unwired: 6 in, 1 out]
        "Buffer Status  (read)" <- w222
        "ReadCircBuf" <- w173
        n142 = Equal?(x=Circular_Buffer_Status."Underflow" ("y"), y=w222) -> (x = y?=→"buffer underflow":bool)
        n143 = Divide(x=w220, y=w219) -> (x/y=w218:dbl)
        n144 = Array Size(array=w173) -> (size(s)=w211:i32)
        n145 = Multiply(x=100.0, y=w218) -> (x*y=→"% buffer full":dbl)
        n146 = Quotient & Remainder(x=w211, y=w183) -> (x-y*floor(x/y)=w210:i32)  [unwired: 1 out]
        n147 = Not Equal To 0?(x=w210) -> (x != 0?=→"non integer read":bool)
        n148 = Search 1D Array(1D array=w173, element=u16 73) -> (index of element=w174:i32)  [unwired: 1 in]
        n149 = Greater Than 0?(x=w174) -> (x > 0?=w175:bool)
        n150 = case shown="True" w175 {
          tunnel: w173 -> [w225 w231]
          tunnel: w174 -> [_ w229]
          tunnel: [w225 w227] -> w172
          frame False {
          }
          frame True {
            n151 = Array Subset(array=w231, index=w229) -> (w226:u16[])  [unwired: 1 in]
            "subReadArray" <- w226
            n152 = call-poly "Circular Buffer.vi"("Read Size"=w229, "Operation"=Circular_Buffer_Operations."Read (continuous)") -> ("Data Out"=w228:u16[])  [unwired: 6 in, 3 out]
            "extrareadelements" <- w228
            n153 = Insert Into Array(array=w226, new element=w228) -> (w227:u16[])  [unwired: 1 in]
            "corrected array" <- w227
            "Nextraadded" <- w229
          }
        }
        n154 = local read "N data scans to read (VISA)"() -> (w180:i32)
        n155 = property on="NumStreamingCluster" class="Clust (strict)"() -> ("Value"=→"ClusterPropnod":T6)  [unwired: 2 in, 2 out]
        n156 = local read "NumStreamingCluster"() -> (w171:T6)
        "ClusterLocalVar" <- w171
        n157 = call "Intan_parseDataStream_128ch.vi"("1-D  data in"=w172, "NumStreamCluster"=w171, "N data scans to read"=w180) -> ("2d ADCdata_array out_ampA_and_B"=w186:u16[][], "Vflex (V) out"=w169:dbl[], "Nscans read"=w201:i32, "aux_cmd_array A"=→"aux_cmd_array":i16[][], "bytes parsed per scan"=→"bytesParsed":i32, "ADXL analog data out"=w189:u16[][], "Vdd (V) out"=w168:dbl[], "MagicNumOut"=→"magicNum Out":i32[])  [unwired: 3 in, 2 out]
        "Vdd (V) out" <- w168
        "Vflex (V) out" <- w169
        n158 = call "ADXL_convert_to_g.vi"("ADXL analog data out: Binary format"=w189) -> ("accelvolts"=w170:dbl[][])  [unwired: 3 in, 1 out]
        n159 = call-poly <vilib>:"Mean.vi"("X"=w168) -> ("mean"=→"Vdd amp (V)":dbl)  [unwired: 1 out]
        n160 = local read "AmpsList"() -> (w181:u16[])
        n161 = local read "ChanSelect"() -> (w182:u16)
        n162 = call "Intan_binary_to_uV.vi"("2d ADC binary data"=w186) -> ("Scaled Data (uV)"=w208:dbl[][])  [unwired: 2 in]
        n163 = property on="Intan Streaming Data" class="WFChart (strict)"() -> ("Plot Bounds"=w207:T9)  [unwired: 2 in, 2 out]
        n164 = local read "YtxtLabelsAll"() -> (w199:string[])
        n165 = Build Array (concatenate)(w170, w169) -> (w167:dbl[][])
        "accel + flex + Vdd array" <- w167
        n166 = Greater Than 0?(x=w201) -> (x > 0?=w212:bool)
        n167 = feedback #3() -> (w185:picture)  [unwired: 1 in]
        n168 = call "Intan_UpdateMarkers_128chan.vi"("Picture In"=w185, "ChanSelectMode"=w182, "Amplifier Chans"=w181, "plot bounds"=w207, "YtxtLabelsAll"=w199) -> ("Picture Out"=w205:picture, "update labels"=w206:bool)
        n169 = feedback-in #3(w205) -> ()
        n170 = case shown="True" w206 {
          tunnel: w205 -> [_ w232]
          frame False {
          }
          frame True {
            n171 = local write "Picture"(w232) -> ()
          }
        }
        n172 = property on="Intan Streaming Data" class="WFChart (strict)"() -> ("XScale.Minimum"=w192:dbl, "XScale.Maximum"=w191:dbl, "XScale.Increment"=w190:dbl)  [unwired: 2 in, 2 out]
        n173 = case shown="True" w212 {
          tunnel: w198 -> [_ w254]
          tunnel: w208 -> [_ w252]
          tunnel: [w233 w245] -> w203
          tunnel: "save aux file" -> [_ w244]
          tunnel: w202 -> [w233 w243]
          tunnel: w201 -> [_ w241]
          tunnel: w192 -> [_ w238]
          tunnel: w191 -> [_ w237]
          tunnel: w190 -> [_ w236]
          tunnel: w167 -> [_ w235]
          frame False {
          }
          frame True {
            # "acceleration vs. time"
            n174 = Unbundle By Name("Filter settings") -> ("LP Filter On/Off"=w250:bool, "HP Filter On/Off"=w249:bool, "Bandstop On/Off"=w247:bool)
            n175 = Compound Arithmetic op=OR("Center Traces", w250, w249, w247) -> (w248:bool)
            n176 = case shown="True" w248 {
              tunnel: w254 -> [_ w334]
              tunnel: w252 -> [w329 w333]
              tunnel: [w329 w332] -> w242
              tunnel: "Filter settings" -> [_ w331]
              tunnel: "Center Traces" -> [_ w330]
              frame False {
              }
              frame True {
                n177 = call "Intan_filter_signals_for_display_v2.vi"("Center Traces"=w330, "input filter cluster"=w331, "Sample Rate (Hz)"=w334, "Nchan Array In [Nchans x Nsamps]"=w333) -> ("Display Signals Out [Nchans x Nsamps]"=w332:dbl[][])
              }
            }
            n178 = property on="DisplayScale (uV/div)" class="Ring (strict)"() -> ("RingText.Text"=w253:string)  [unwired: 2 in, 2 out]
            n179 = Decimal String To Number(string=w253) -> (number=w255:i32)  [unwired: 2 in, 1 out]
            n180 = call "Intan_binary_to_uV_offset_and_scale.vi"("offset spacing factor"="offset factor", "Yscale (uv/div)"=w255, "ScaledData [Nchans x Nsamps]"=w242) -> ("Nchannels"=w239:i32, "Data4Display"=w234:dbl[][])  [unwired: 1 in]
            n181 = stacked-sequence {
              tunnel: w241 -> [_ w280]
              tunnel: "offset factor" -> [_ w267]
              tunnel: w239 -> [_ w260]
              tunnel: w238 -> [_ w263]
              tunnel: w237 -> [_ w262]
              tunnel: w236 -> [_ w261]
              tunnel: w235 -> [w258 _]
              tunnel: w234 -> [w257 _]
              frame #0 {
                # "force updates between 2 plots to happen at same time"
                n182 = Array Size(array=w258) -> (size(s)=→"adxl size":i32[])
                n183 = Array Size(array=w257) -> (size(s)=→"intan size":i32[])
                "ADXL/Vflex/Vdd Stream" <- w258
                "Intan Streaming Data" <- w257
              }
              frame #1 {
                # "update axes as needed"
                # "update axes depending on\non-the-fly  user settings"
                n184 = local read "increment_init"() -> (w266:dbl)
                n185 = local read "ChartDisplayLength (s)"() -> (w278:dbl)
                n186 = local read "DT_scale (sec)"() -> (w277:dbl)
                n187 = local read "FS (Hz)"() -> (w279:dbl)
                n188 = Bundle("XScale.Minimum"=w263, "XScale.Maximum"=w262, "XScale.Increment"=w261, "Nchannels"=w260) -> (w264:T11)  [unwired: 1 in]
                n189 = call "Intan_Update_XY_AxisLims.vi"("NscansRead"=w280, "offset factor"=w267, "FS (Hz)"=w279, "XscaleClusterCurrent"=w264, "DisplayLength(s)"=w278, "DT_scale (s)"=w277) -> ("XscaleRollover"=→"XscaleRollover":bool, "DispLengthChanged"=→"DispLengthChanged":bool, "NchansChanged"=→"NchansChanged":bool, "XYlims Update Cluster"=w275:T12, "UpdateCode"=w276:i16)  [unwired: 4 in, 1 out]
                "UpdateCode" <- w276
                n190 = Unbundle(w275) -> ("Maximum"=w272:dbl, w271:dbl, w269:dbl, w268:dbl, w274:dbl, w273:dbl, "YscleMark"=w270:dbl)  [unwired: 1 out]
                n191 = case shown="0, Default" w276 {
                  tunnel: w260 -> [_ _ _ w300 w311]
                  tunnel: w274 -> [_ _ _ w295 _]
                  tunnel: w273 -> [_ _ _ w299 _]
                  tunnel: w272 -> [_ w285 _ _ w314]
                  tunnel: w271 -> [_ w284 _ _ w313]
                  tunnel: w270 -> [_ _ _ w298 w312]
                  tunnel: w269 -> [_ _ w290 _ _]
                  tunnel: w268 -> [_ _ w291 _ _]
                  tunnel: w267 -> [_ _ _ w297 w310]
                  tunnel: w266 -> [_ w283 w289 w296 w309]
                  frame 0, Default {
                    # "nothing to update"
                  }
                  frame 1 {
                    # "normal X axis rollover"
                    n192 = stacked-sequence {
                      tunnel: w285 -> [w286 _ _]
                      tunnel: w284 -> [_ w287 _]
                      tunnel: w283 -> [_ _ w288]
                      frame #0 {
                        n193 = property on="Intan Streaming Data" class="WFChart (strict)"("XScale.Minimum"=w286) -> ()  [unwired: 2 in, 2 out]
                        n194 = property on="ADXL/Vflex/Vdd Stream" class="WFChart (strict)"("XScale.Minimum"=w286) -> ()  [unwired: 2 in, 2 out]
                      }
                      frame #1 {
                        n195 = property on="Intan Streaming Data" class="WFChart (strict)"("XScale.Maximum"=w287) -> ()  [unwired: 2 in, 2 out]
                        n196 = property on="ADXL/Vflex/Vdd Stream" class="WFChart (strict)"("XScale.Maximum"=w287) -> ()  [unwired: 2 in, 2 out]
                      }
                      frame #2 {
                        n197 = property on="Intan Streaming Data" class="WFChart (strict)"("XScale.Increment"=w288) -> ()  [unwired: 2 in, 2 out]
                        n198 = property on="ADXL/Vflex/Vdd Stream" class="WFChart (strict)"("XScale.Increment"=w288) -> ()  [unwired: 2 in, 2 out]
                      }
                    }
                  }
                  frame 2 {
                    # "updated display length"
                    n199 = stacked-sequence {
                      tunnel: w289 -> [_ _ w294]
                      tunnel: w291 -> [_ w293 _]
                      tunnel: w290 -> [w292 _ _]
                      frame #0 {
                        n200 = property on="Intan Streaming Data" class="WFChart (strict)"("XScale.Minimum"=w292) -> ()  [unwired: 2 in, 2 out]
                        n201 = property on="ADXL/Vflex/Vdd Stream" class="WFChart (strict)"("XScale.Minimum"=w292) -> ()  [unwired: 2 in, 2 out]
                      }
                      frame #1 {
                        n202 = property on="Intan Streaming Data" class="WFChart (strict)"("XScale.Maximum"=w293) -> ()  [unwired: 2 in, 2 out]
                        n203 = property on="ADXL/Vflex/Vdd Stream" class="WFChart (strict)"("XScale.Maximum"=w293) -> ()  [unwired: 2 in, 2 out]
                      }
                      frame #2 {
                        n204 = property on="Intan Streaming Data" class="WFChart (strict)"("XScale.Increment"=w294) -> ()  [unwired: 2 in, 2 out]
                        n205 = property on="ADXL/Vflex/Vdd Stream" class="WFChart (strict)"("XScale.Increment"=w294) -> ()  [unwired: 2 in, 2 out]
                      }
                    }
                  }
                  frame 3 {
                    # "update N chans display"
                    n206 = stacked-sequence {
                      tunnel: w300 -> [w304 _ _ _ _]
                      tunnel: w296 -> [_ _ _ _ w308]
                      tunnel: w299 -> [_ _ _ w307 _]
                      tunnel: w298 -> [_ _ _ _ _]
                      tunnel: w297 -> [w302 _ _ _ _]
                      tunnel: w295 -> [_ w305 w306 _ _]
                      frame #0 {
                        n207 = Negate(x=w304) -> (-x=w303:i32)
                        n208 = Multiply(x=w302, y=w303) -> (x*y=w301:dbl)
                        n209 = property on="Intan Streaming Data" class="WFChart (strict)"("YScale.Minimum"=w301) -> ()  [unwired: 2 in, 2 out]
                      }
                      frame #1 {
                        n210 = property on="Intan Streaming Data" class="WFChart (strict)"("XScale.Offset"=w305) -> ()  [unwired: 2 in, 2 out]
                      }
                      frame #2 {
                        n211 = property on="Intan Streaming Data" class="WFChart (strict)"("XScale.Minimum"=w306) -> ()  [unwired: 2 in, 2 out]
                      }
                      frame #3 {
                        n212 = property on="Intan Streaming Data" class="WFChart (strict)"("XScale.Maximum"=w307) -> ()  [unwired: 2 in, 2 out]
                      }
                      frame #4 {
                        n213 = property on="Intan Streaming Data" class="WFChart (strict)"("XScale.Increment"=w308) -> ()  [unwired: 2 in, 2 out]
                      }
                    }
                  }
                  frame 4 {
                    # "updated offset factor"
                    n214 = stacked-sequence {
                      seq-local: [w315 _ _] -> [_ w319 _]
                      tunnel: w314 -> [_ _ _]
                      tunnel: w313 -> [_ _ _]
                      tunnel: w312 -> [_ _ _]
                      tunnel: w311 -> [w318 _ _]
                      tunnel: w310 -> [w316 _ _]
                      tunnel: w309 -> [_ _ w324]
                      frame #0 {
                        n215 = Negate(x=w318) -> (-x=w317:i32)
                        n216 = Multiply(x=w316, y=w317) -> (x*y=w315:dbl)
                        n217 = property on="Intan Streaming Data" class="WFChart (strict)"("YScale.Minimum"=w315) -> ()  [unwired: 2 in, 2 out]
                      }
                      frame #1 {
                        n218 = for {
                          N: w319 -> [_]
                          tunnel: [w322] -> w321 mode=indexing
                          i -> [w323]
                          n219 = Negate(x=w323) -> (-x=w322:i32)
                        }
                        n220 = To Double Precision Float(number=w321) -> (double precision float=w320:dbl[])
                        n221 = property on="Intan Streaming Data" class="WFChart (strict)" props=["YScale", "MarkerVals[]", "YScale", "MarkerVals[]"]("YScale.MarkerVals[]"=w320) -> ()  [unwired: 2 in, 3 out]
                      }
                      frame #2 {
                        n222 = property on="Intan Streaming Data" class="WFChart (strict)"("XScale.Increment"=w324) -> ()  [unwired: 2 in, 2 out]
                      }
                    }
                  }
                }
              }
            }
            n223 = case shown="False" w244 {
              tunnel: w234 -> [_ w328]
              tunnel: [w325 w327] -> w245
              tunnel: w243 -> [w325 w326]
              frame False {
              }
              frame True {
                n224 = call "Intan_SaveDisplayData.vi"("2d ADCdata_array out"=w328, "aux file ref num"=w326) -> ("refnum out"=w327:refnum<file>)  [unwired: 3 in]
              }
            }
          }
        }
        n225 = local read "StopLoopsMaster"() -> (w200:bool)
        "display iter" <- w214
      }
    }
    frame #4 {
      w503 = u16 2 items=["None", "Last Bit", "TermChar"] ("Serial Settings:End Mode for Reads")
      # "There may still be some bytes waiting from last serial.write\nafter the 'p' char is sent to Teensy. Clearing the port just makes\nit more likely we see the Teensy response text response to 'p' \nby getting rid of 'extra' data bytes waiting"
      # "After user terminates acquisition (or error), need to:\n- write 'q' to Teensy to pause serial writes. Note: SPI/ADC converts + writing to SD card continues for ambulatory system\n- close VISA session\n- close LV data file\nNote we turn term char en = true so we can read out user friendly text after pausing"
      n226 = local read "Save Binary Data"() -> (w490:bool)
      n227 = case shown="False" w491 {
        tunnel: w493 -> [_ w514]
        frame False {
        }
        frame True {
          n228 = Close File(refnum=w514) -> ()  [unwired: 1 in, 2 out]
        }
      }
      n229 = property class="Serial Instr"(reference=w498, error in=w492, "TermChar En"=TRUE ("Message Based Settings:Termination Character Enable"), "ASRL End In"=w503) -> (reference out=w497:refnum<visa-resource-name>, error out=w496:errorcluster)
      n230 = case shown="False" w490 {
        tunnel: w511 -> [_ w512]
        frame False {
        }
        frame True {
          n231 = Close File(refnum=w512) -> (error out=w513:errorcluster)  [unwired: 1 in, 1 out]
          n232 = call <vilib>:"Simple Error Handler.vi"("error in (no error)"=w513) -> ()  [unwired: 4 in, 5 out]
        }
      }
      n233 = VISA Clear(VISA resource name=w497, error in (no error)=w496) -> (VISA resource name out=w495:refnum<visa-resource-name>, error out=w494:errorcluster)
      n234 = VISA Write(VISA resource name=w495, write buffer="stop serial stream (Teensy char)", error in (no error)=w494) -> (VISA resource name out=w506:refnum<visa-resource-name>, error out=w505:errorcluster)  [unwired: 1 out]
      n235 = VISA Read(VISA resource name=w506, byte count=u32 20000, error in (no error)=w505) -> (VISA resource name out=w502:refnum<visa-resource-name>, read buffer=→"Text response":string, error out=w500:errorcluster)  [unwired: 1 out]
      n236 = VISA Clear(VISA resource name=w502, error in (no error)=w500) -> (VISA resource name out=w501:refnum<visa-resource-name>, error out=w499:errorcluster)
      n237 = VISA Close(VISA resource name=w501, error in (no error)=w499) -> (error out=→"error out":errorcluster)
    }
  }
